vi "RecordingPath.vi"(8 "error in (no error)":errorcluster, 9 "Extension":string, 10 "Recording Root":path=path "C:/temp.tdms", 11 "AcquistionObject in":refnum<class "AcquistionObject.lvclass">) -> (0 "error out":errorcluster, 2 "FilePath":path, 3 "AcquistionObject out":refnum<class "AcquistionObject.lvclass">)   [LabVIEW 2010, in "AcquistionObject.lvclass"]
uses:
  AcquistionObject.lvclass
  AcquistionObject.lvclass/AcquistionObject.ctl
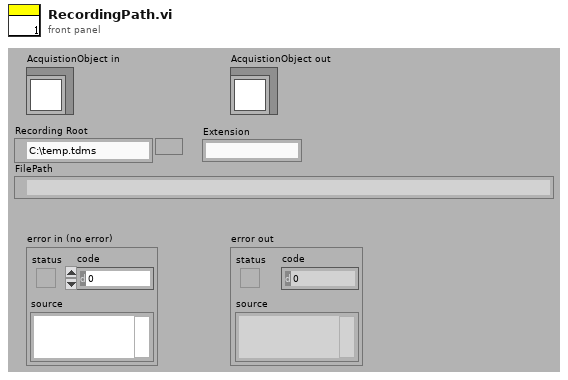
[diagram p1: front panel]
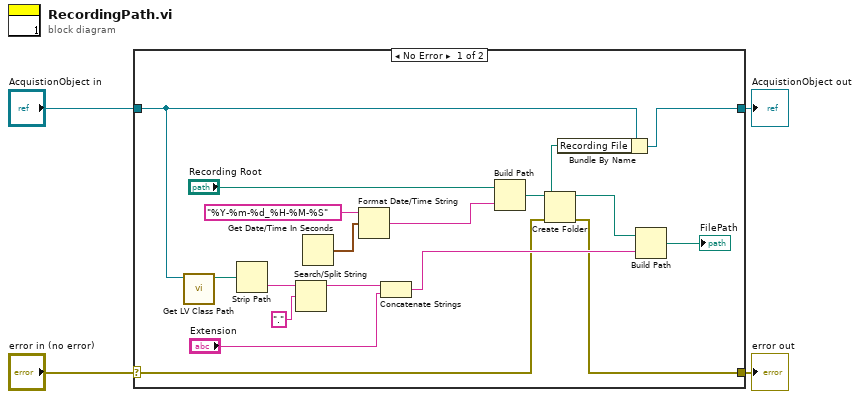
[diagram p0: block diagram]
diagram:
  n1 = case shown="No Error" "error in (no error)" {
    selector: "error in (no error)" -> [w6 w23]
    tunnel: [w5 w23] -> w3
    tunnel: [w12 w22] -> w1
    tunnel: "AcquistionObject in" -> [w13 w22]
    frame No Error {
      n2 = call <vilib>:"Get LV Class Path.vi"("object"=w13) -> ("class path"=w18:path)  [unwired: 9 in, 1 out]
      n3 = Strip Path(path=w18) -> (name=w17:string)  [unwired: 1 out]
      n4 = Search/Split String(string=w17, search string/char (-)=".") -> (substring before match=w15:string)  [unwired: 1 in, 2 out]
      n5 = Get Date/Time In Seconds() -> (seconds since 1Jan1904=w19:timestamp)
      n6 = Format Date/Time String(time format string (%c)="%Y-%m-%d_%H-%M-%S", seconds (now)=w19) -> (date/time string=w11:string)  [unwired: 1 out]
      n7 = Concatenate Strings(w15, "Extension") -> (w10:string)
      n8 = Build Path(base path="Recording Root", name or relative path=w11) -> (appended path=w8:path)
      n9 = Create Folder(path (use dialog)=w8, error in=w6) -> (created path=w7:path, error out=w5:errorcluster)  [unwired: 1 in, 1 out]
      n10 = Bundle By Name(cluster=w13, "Recording File"=w8) -> (w12:refnum<class "AcquistionObject.lvclass">)
      n11 = Build Path(base path=w7, name or relative path=w10) -> (appended path=→"FilePath":path)
    }
    frame Error {
    }
  }
  "error out" <- w3
  "AcquistionObject out" <- w1
